vi "svfa_Get Frequencies for LabVIEW Double-Sided FFT.vi"(7 "frequency units":u16(ring)=2 items=["cycles per second (Hz)", "radians per second (rad/s)", "cycles per sample"], 9 "shift":bool, 10 "dt":dbl=0.001, 11 "FFT length":i32=1000) -> (2 "df":dbl=nan, 3 "spectrum frequencies":dbl[](graph))   [LabVIEW 2017]
uses:
  <vilib>/Analysis/1siggen.llb/Ramp Pattern by Samples.vi
  <vilib>/Analysis/NI_AALBase.lvlib
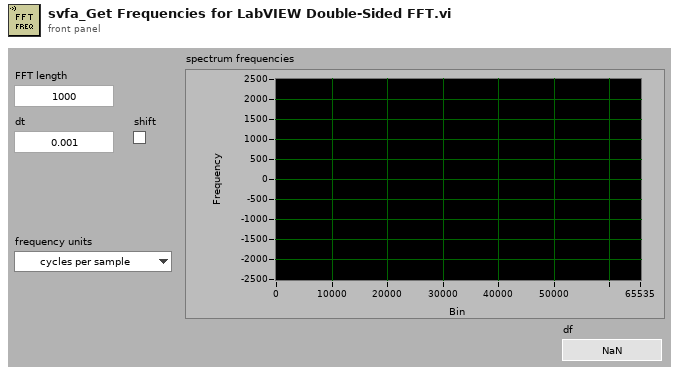
[diagram p1: front panel]
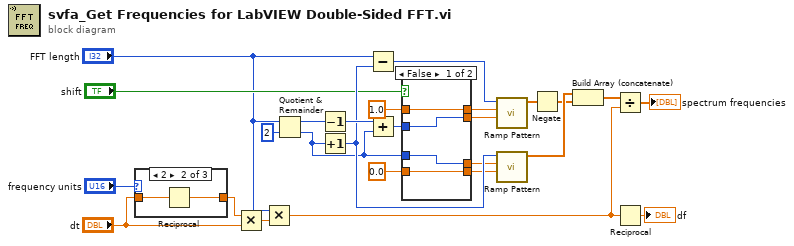
[diagram p0: block diagram]
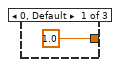
[diagram p2: hidden frame]
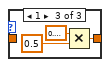
[diagram p3: hidden frame]
diagram:
  n1 = case shown="2" "frequency units" {
    tunnel: "dt" -> [_ w29 _]
    tunnel: [1.0 ("value") w28 w31] -> w4
    frame 0, Default {
    }
    frame 2 {
      n2 = Reciprocal(x=w29) -> (1/x=w28:dbl)
    }
    frame 1 {
      n3 = Multiply(x=0.3183098861837907, y=0.5 ("x")) -> (x*y=w31:dbl)
    }
  }
  n4 = Multiply(x=w4, y="dt") -> (x*y=w6:dbl)
  n5 = Multiply(x="FFT length", y=w6) -> (x*y=w1:dbl)
  n6 = Quotient & Remainder(x="FFT length", y=2) -> (x-y*floor(x/y)=w23:i32, floor(x/y)=w13:i32)
  n7 = Decrement(x=w23) -> (x-1=w22:i32)
  n8 = Increment(x=w13) -> (x+1=w15:i32)
  n9 = Subtract(x="FFT length", y=w15) -> (x-y=w24:i32)
  n10 = Add(x=w22, y=w13) -> (x+y=w19:i32)
  n11 = case shown="False" "shift" {
    tunnel: [w36 w40] -> w18
    tunnel: w19 -> [w36 w39]
    tunnel: [w35 w39] -> w16
    tunnel: 1.0 ("start") -> [w35 w40]
    tunnel: [w34 w37] -> w14
    tunnel: w13 -> [w34 w38]
    tunnel: [w33 w38] -> w12
    tunnel: 0.0 ("start") -> [w33 w37]
    frame False {
    }
    frame True {
    }
  }
  n12 = call-poly <vilib>:"Ramp Pattern.vi"("start"=w18, "end"=w16, "samples"=w24) -> ("Ramp Pattern"=w21:dbl[])  [unwired: 7 in, 1 out]
  n13 = call-poly <vilib>:"Ramp Pattern.vi"("start"=w12, "end"=w14, "samples"=w15) -> ("Ramp Pattern"=w20:dbl[])  [unwired: 7 in, 1 out]
  n14 = Negate(x=w21) -> (-x=w8:dbl[])
  n15 = Build Array (concatenate)(w20, w8) -> (w25:dbl[])
  n16 = Divide(x=w25, y=w1) -> (x/y=→"spectrum frequencies":dbl[])
  n17 = Reciprocal(x=w1) -> (1/x=→"df":dbl)
